vi "Main Loop.vi"(8 "error in (no error)":errorcluster, 10 "Chart Notifier":refnum<notifier>, 11 "Message Queues":T1) -> (0 "error out":errorcluster)   [LabVIEW 2018, in "4-20mA Module.lvlib" / "4-20mA Module Engine.lvlib"]
uses:
  4-20mA Module Engine.lvlib
  Pressure Regulator/Controls/4-20mA Message Queues.ctl
  support/Message Queue/Message Cluster.ctl
  State Cluster.ctl
  State Enum.ctl
  Pressure Transmitter/Pressure Transmitter Device Settings.ctl
  Pressure Reg Module/Pressure Regulator Device Settings.ctl
  Measure Instrument/PID 1 Parameters Cluster.ctl
  Pressure Regulator/Controls/4-20mA Display Cluster.ctl
  <vilib>/Platform/TimedLoop/XDataNode/timing_clust.ctl
  <vilib>/Platform/TimedLoop/XDataNode/nitl_modes.ctl
  <vilib>/Platform/TimedLoop/XDataNode/wakeup.ctl
  Tag VIs/Tag FGV Operation Enum.ctl
  Pressure Regulator/Controls/4-20mA Module Settings Cluster.ctl
  support/Message Queue/Enqueue Message (Single).vi
  <vilib>/Platform/TimedLoop/XDataNode/XDataNode.xnode
  support/Message Queue/Message Queue.lvlib
  <vilib>/Platform/TimedLoop/XDataNode/XDNodeRunTimeDep.lvlib
  Shared Variables/Dynamic Shared Variables.lvlib
  Pressure Transmitter/Pressure Transmitter Library.lvlib
  Pressure Reg Module/Pressure Regulator Library.lvlib
  Pressure Regulator/4-20mA Module.lvlib
  support/Support Library.lvlib
panel:
  out "Period (s)":dbl format="%_4g"
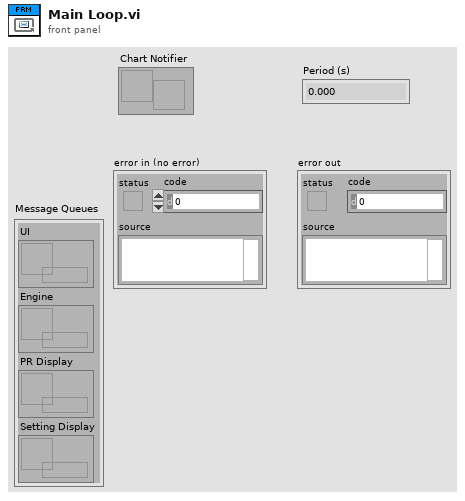
[diagram p1: front panel]
types:
  T1 = typedef "4-20mA Module.lvlib/4-20mA Message Queues.ctl" = cluster{"UI":refnum<queue>, "Engine":refnum<queue>, "PR Display":refnum<queue>, "Setting Display":refnum<queue>}
  T2 = typedef "4-20mA Module.lvlib/4-20mA Display Cluster.ctl" = cluster{"Input 4-20":dbl, "Output 4-20":dbl, "Cycle Period":dbl, "Status":enum16{"Off", "On", "Not Initialized"}}
  T3 = typedef "XDNodeRunTimeDep.lvlib/timing_clust.ctl" = cluster{"Expected End [f-1]":u64, "Actual End [f-1]":u64, "Finished Late? [f-1]":bool, "Expected End [i-1]":u64, "Actual End [i-1]":u64, "Finished Late? [i-1]":bool, "Expected Start [i]":u64, "Actual Start [i]":u64, "Expected Start [f]":u64, "Actual Start [f]":u64, "Source Name":string, "Structure Name":string, "Period":i64, "Deadline":i64, "Offset":i64, "Start":i64, "Priority":i32, "Timeout":i32, "Mode":T4, "Wakeup Reason":T5, "Error":errorcluster, "Source Type":string, "Secondary Source Type":string, "Global End Time":u64, "Global Start Time":u64, "Frame Duration":u64, "Iteration Duration":u64, "Assigned CPU":i32, "I/O Scan Engine Mode":u32}
  T4 = typedef "XDNodeRunTimeDep.lvlib/nitl_modes.ctl" = enum32{"No Change", "Process missed periods, maintain original phase", "Discard missed periods, maintain original phase", "Process missed periods, ignore original phase", "Discard missed periods, ignore original phase"}
  T5 = typedef "XDNodeRunTimeDep.lvlib/wakeup.ctl" = enum32{"Normal", "Aborted", "Asynchronous wakeup", "Timing source error", "Timed loop error", "Timeout"}
  T6 = cluster{"enable? (F)":bool, "name":string, "alarm on":bool, "priority":u32, "ack type":enum16{"Auto", "User", "None", "Each Occurrence"}, "area":string, "description":string, "log? (T)":bool}
  T7 = typedef "Tag FGV Operation Enum.ctl" = enum16{"Init", "Set Notification Queue", "Create Tag", "Commit", "Write Tag (Numeric)", "Write Tag (Boolean)", "Read All Tags", "Read One Tag", "Delete Tag Category", "Set Alarm Parameters (Numeric)", "Set Alarm Parameters (Boolean)", "Enable All Alarms", "Disable All Alarms", "Delete All Tags", "Read Alarms", "Ack Alarm", "Read Alarm Parameters (Numeric)", "Read Alarm Parameters (Boolean)"}
  T8 = enum32{"u32BitField", "bool", "double", "string", "int8", "uint8", "int16", "uint16", "int32", "uint32", "int64", "uint64", "single", "double waveform", "int16 waveform", "array of boolean", "array of int8", "array of uint8", "array of int16", "array of uint16", "array of int32", "array of uint32", "array of int64", "array of uint64", "array of single", "array of double", "array of double waveform", "array of int16 waveform", "array of string", "variant", "timestamp", "fixed point", "custom"}
  T9 = typedef "4-20mA Module.lvlib/4-20mA Module Engine.lvlib/State Enum.ctl" = enum16{"Measuring", "Idle", "Paused"}
  T10 = typedef "4-20mA Module.lvlib/4-20mA Module Settings Cluster.ctl" = cluster{"Cycle Period":dbl, "PID 2 Parameters":cluster{"Input Device":enum16{"Default", "4-20mA"}, "Output Device":enum16{"Default", "Equilibar Pressure Reg", "Flow Regulator"}, "Setpoint":dbl, "PID gains":cluster{"proportional gain (Kc)":dbl, "integral time (Ti, min)":dbl, "derivative time (Td, min)":dbl}, "output range":cluster{"output low":dbl, "output high":dbl}}, "Manual Entry":dbl, "Auto?":bool, "4-20mA Input Settings":T11, "4-20mA Out Settings":T12, "Input Channel Tag Name ":string}
  T11 = typedef "Pressure Transmitter Library.lvlib/Pressure Transmitter Device Settings.ctl" = cluster{"Input Channel ":u16}
  T12 = typedef "Pressure Regulator Library.lvlib/Pressure Regulator Device Settings.ctl" = cluster{"Output DAQ Task":refnum<k21>}
  T13 = typedef "4-20mA Module.lvlib/4-20mA Module Engine.lvlib/State Cluster.ctl" = cluster{"State":T9, "Start Time":timestamp, "Configuration":cluster{"Cycle Period":dbl, "PID 2 Parameters":cluster{"Input Device":enum16{"Default", "4-20mA"}, "Output Device":enum16{"Default", "Equilibar Pressure Reg", "Flow Regulator"}, "Setpoint":dbl, "PID gains":cluster{"proportional gain (Kc)":dbl, "integral time (Ti, min)":dbl, "derivative time (Td, min)":dbl}, "output range":cluster{"output low":dbl, "output high":dbl}}, "Manual Entry":dbl, "Auto?":bool, "4-20mA Input Settings":T11, "4-20mA Out Settings":T12, "Input Channel Tag Name ":string}, "Current Time":timestamp, "PID 1 Parameters":T14, "First Iteration":bool, "Data":cluster{"4-20mA Input":dbl, "PID 2 Process Variable":dbl, "PID 2 Output":dbl, "4-20mA Output":dbl}, "Process Name":string, "Pump On?":enum16{"Off", "On", "Not Initialized"}, "Input Error":bool, "Output Error":bool, "Log Started":bool, "Current Setpoint":dbl}
  T14 = typedef "PID 1 Parameters Cluster.ctl" = cluster{"Setpoint":dbl, "PID gains":cluster{"proportional gain (Kc)":dbl, "integral time (Ti, min)":dbl, "derivative time (Td, min)":dbl}}
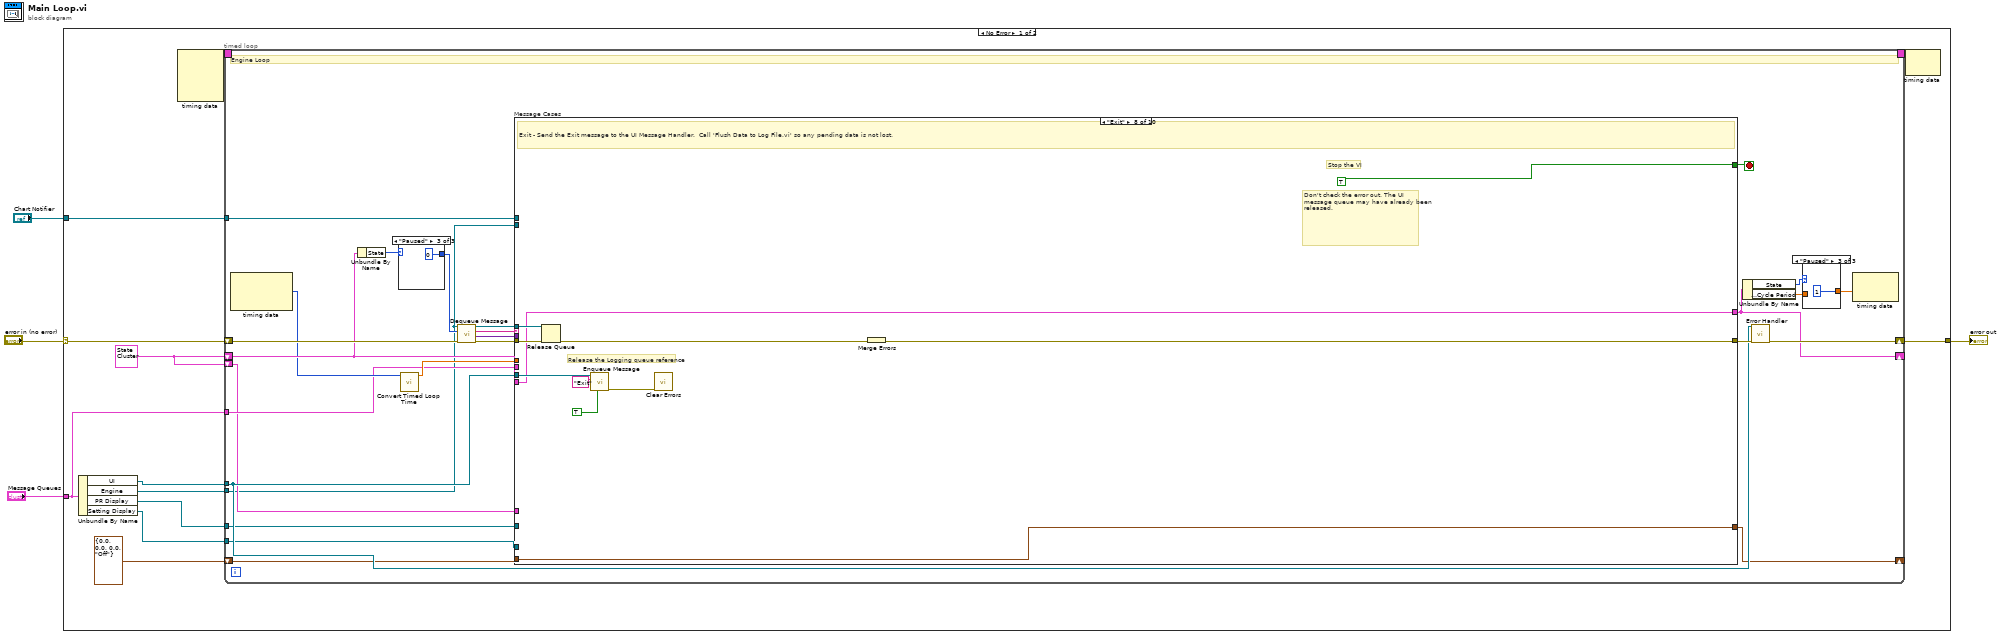
[diagram p0: block diagram]
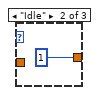
[diagram p3: hidden frame]
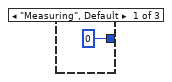
[diagram p4: hidden frame]
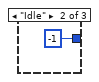
[diagram p5: hidden frame]
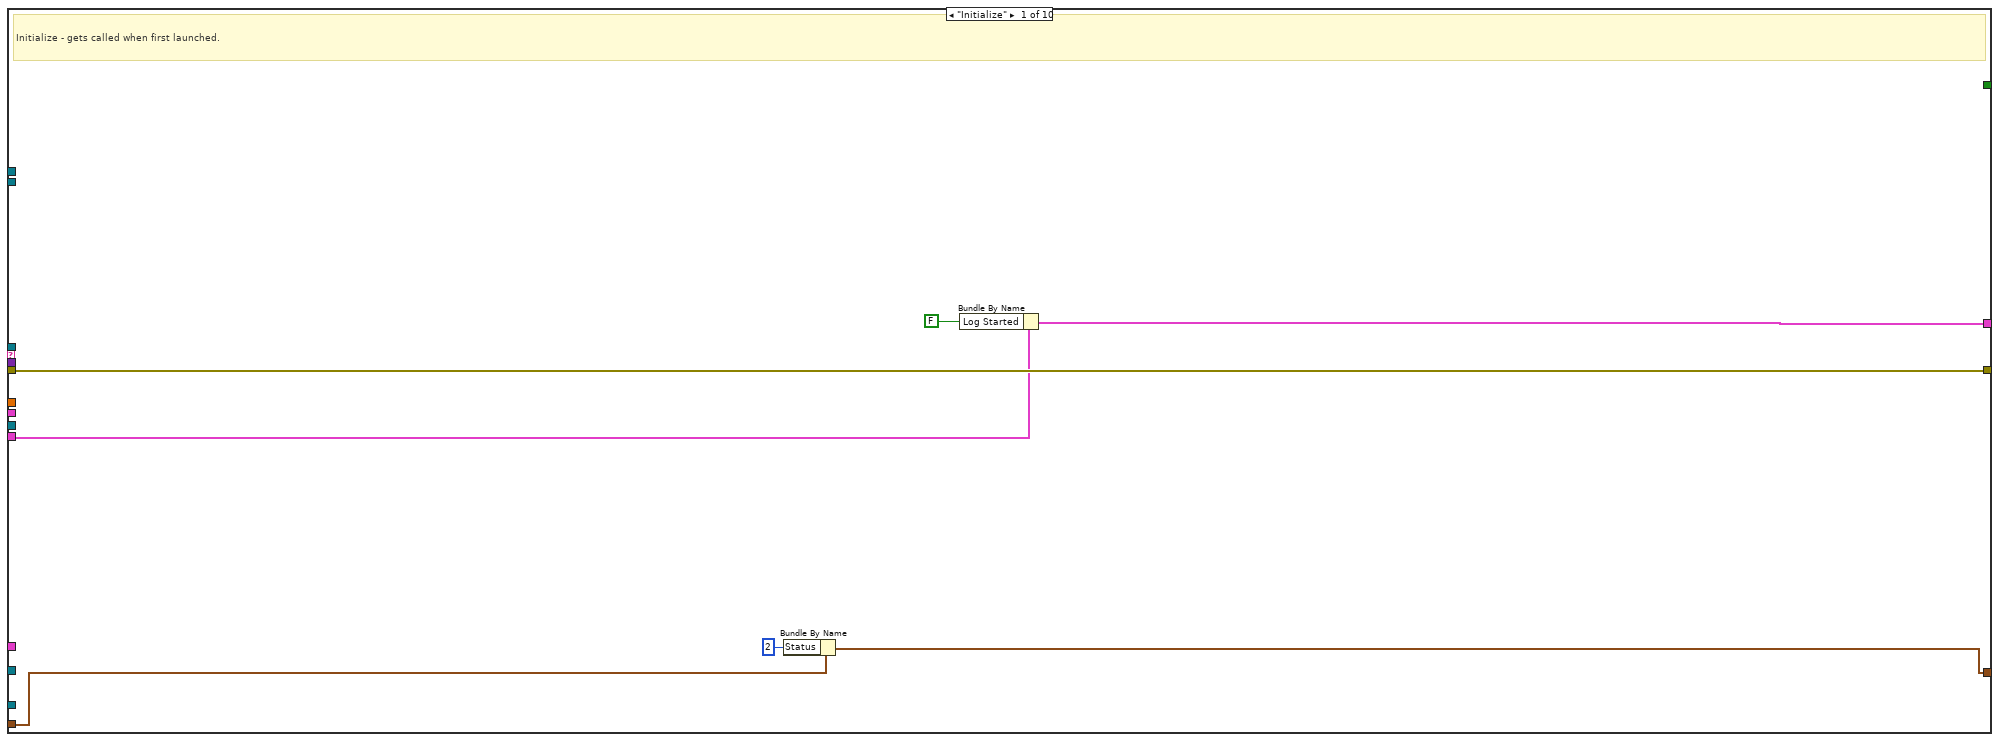
[diagram p6: hidden frame]
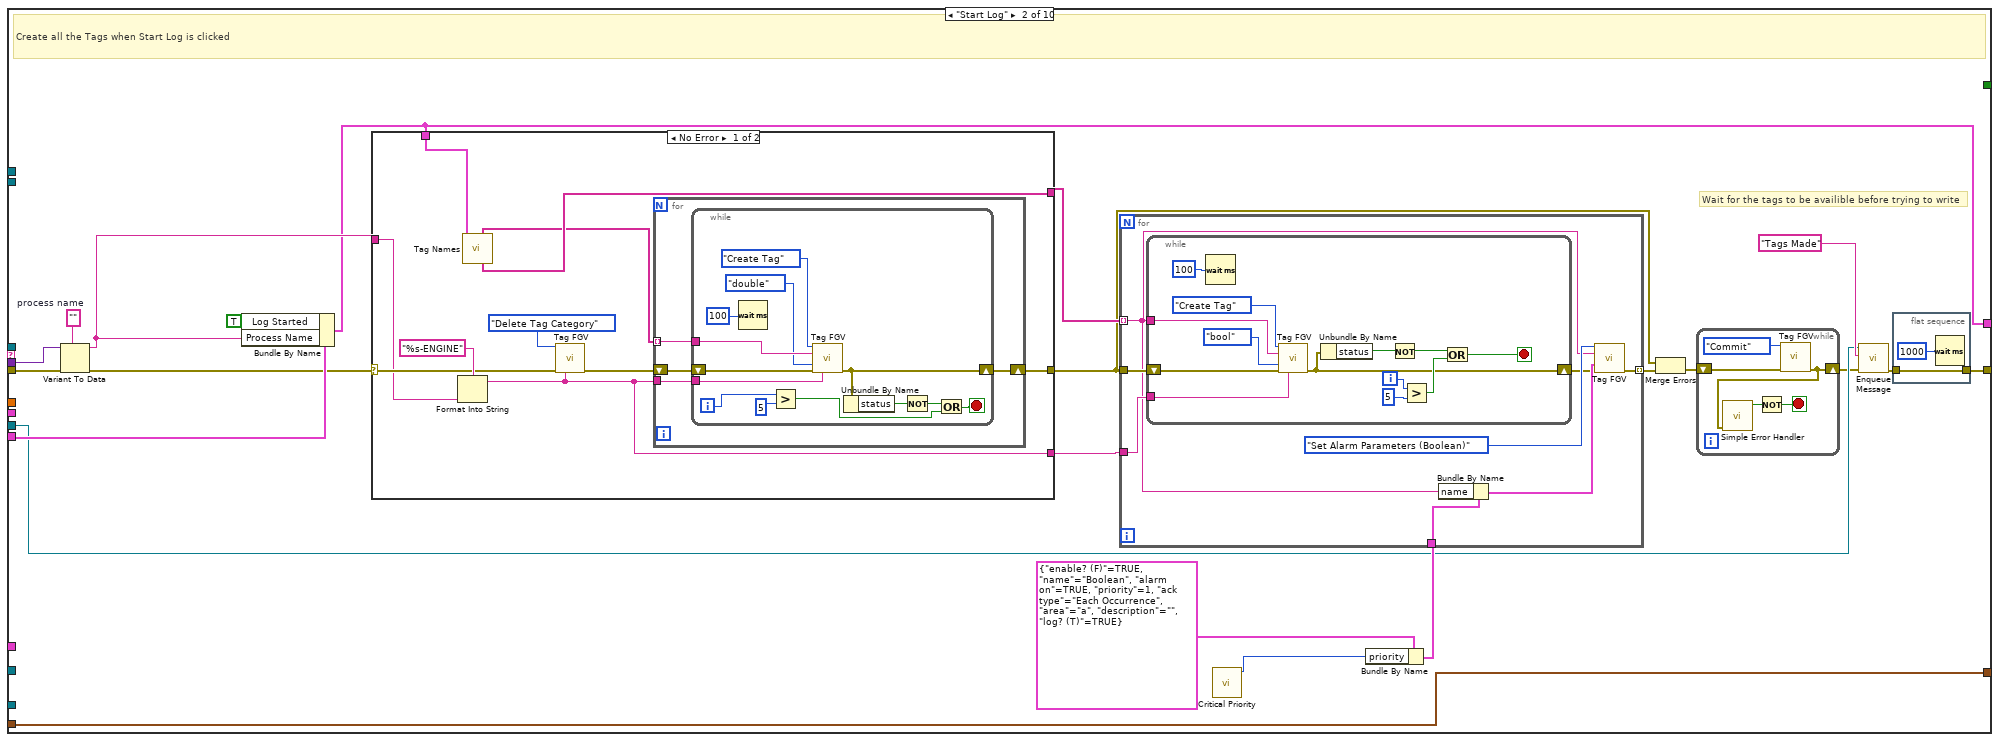
[diagram p7: hidden frame]
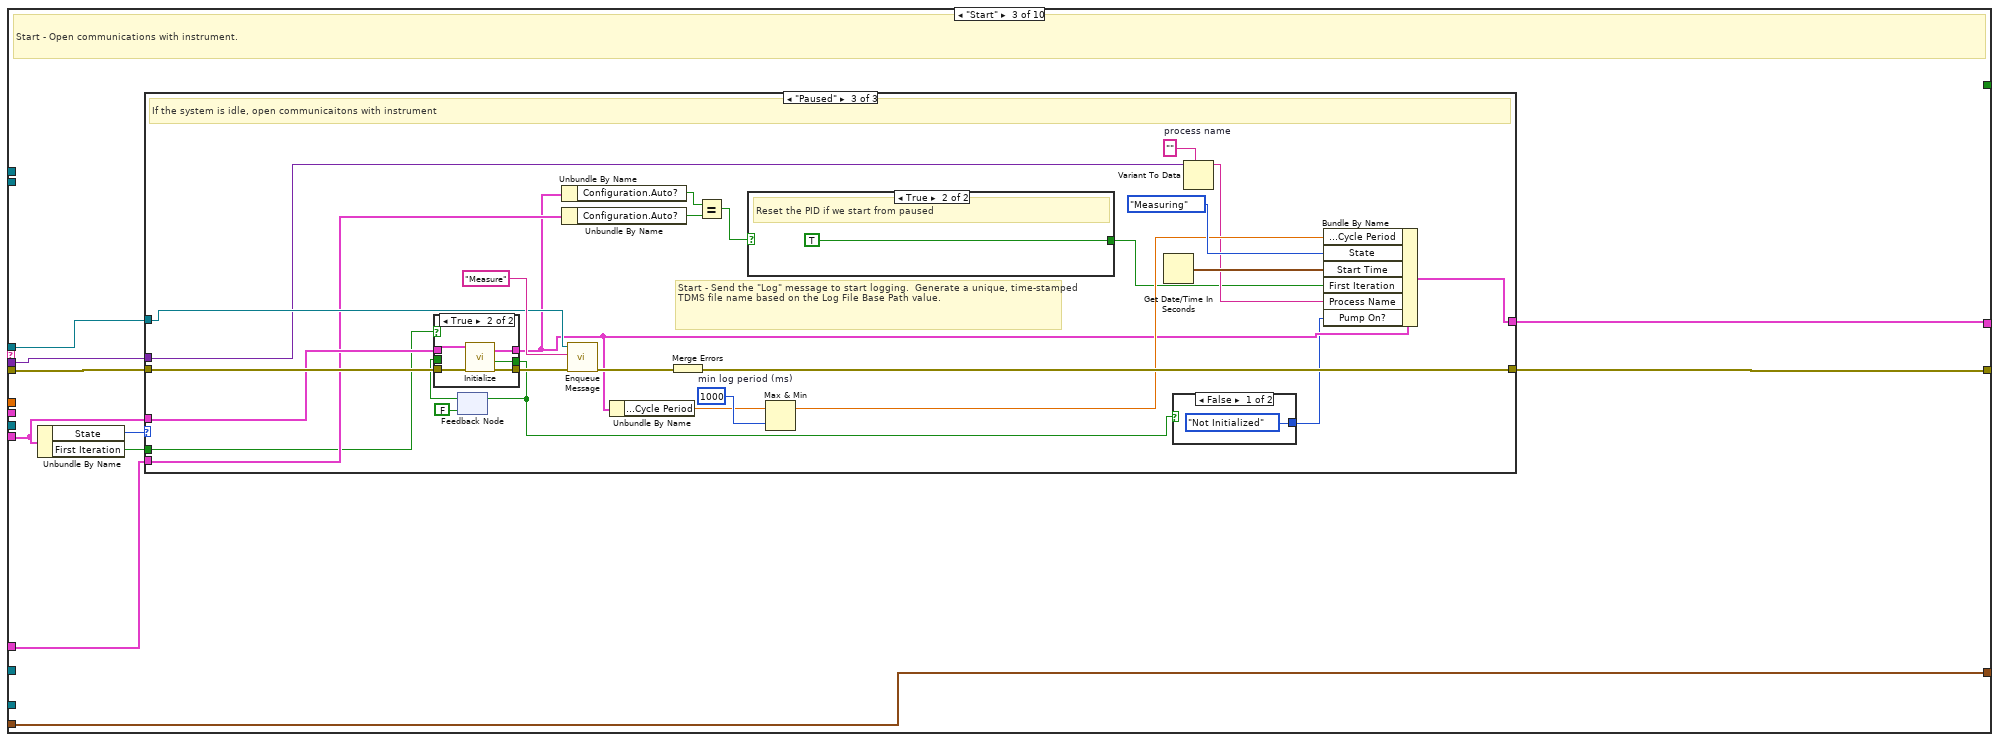
[diagram p9: hidden frame]
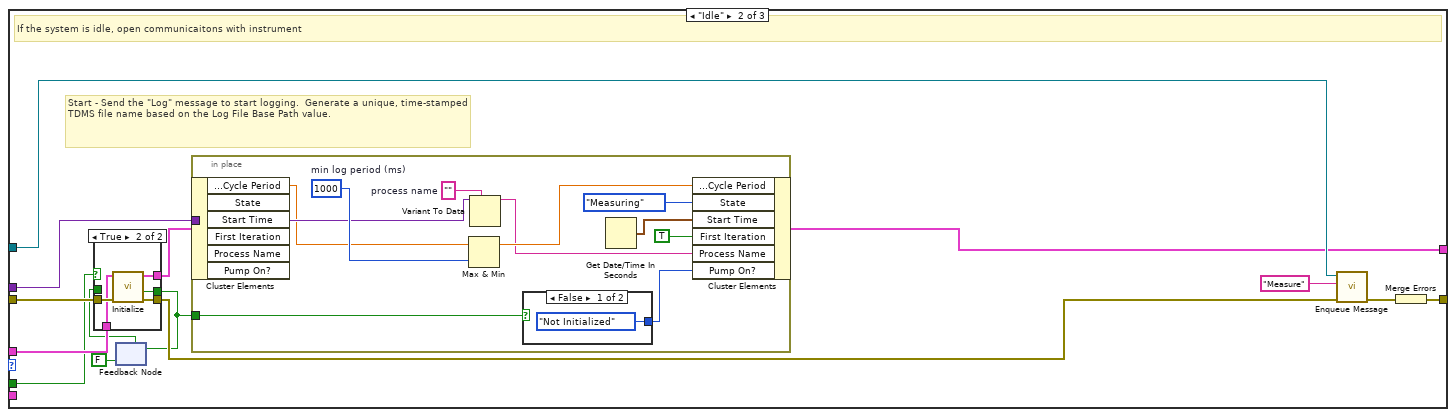
[diagram p11: hidden frame]
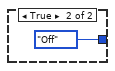
[diagram p12: hidden frame]
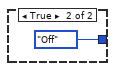
[diagram p15: hidden frame]
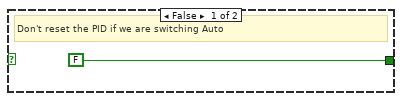
[diagram p16: hidden frame]
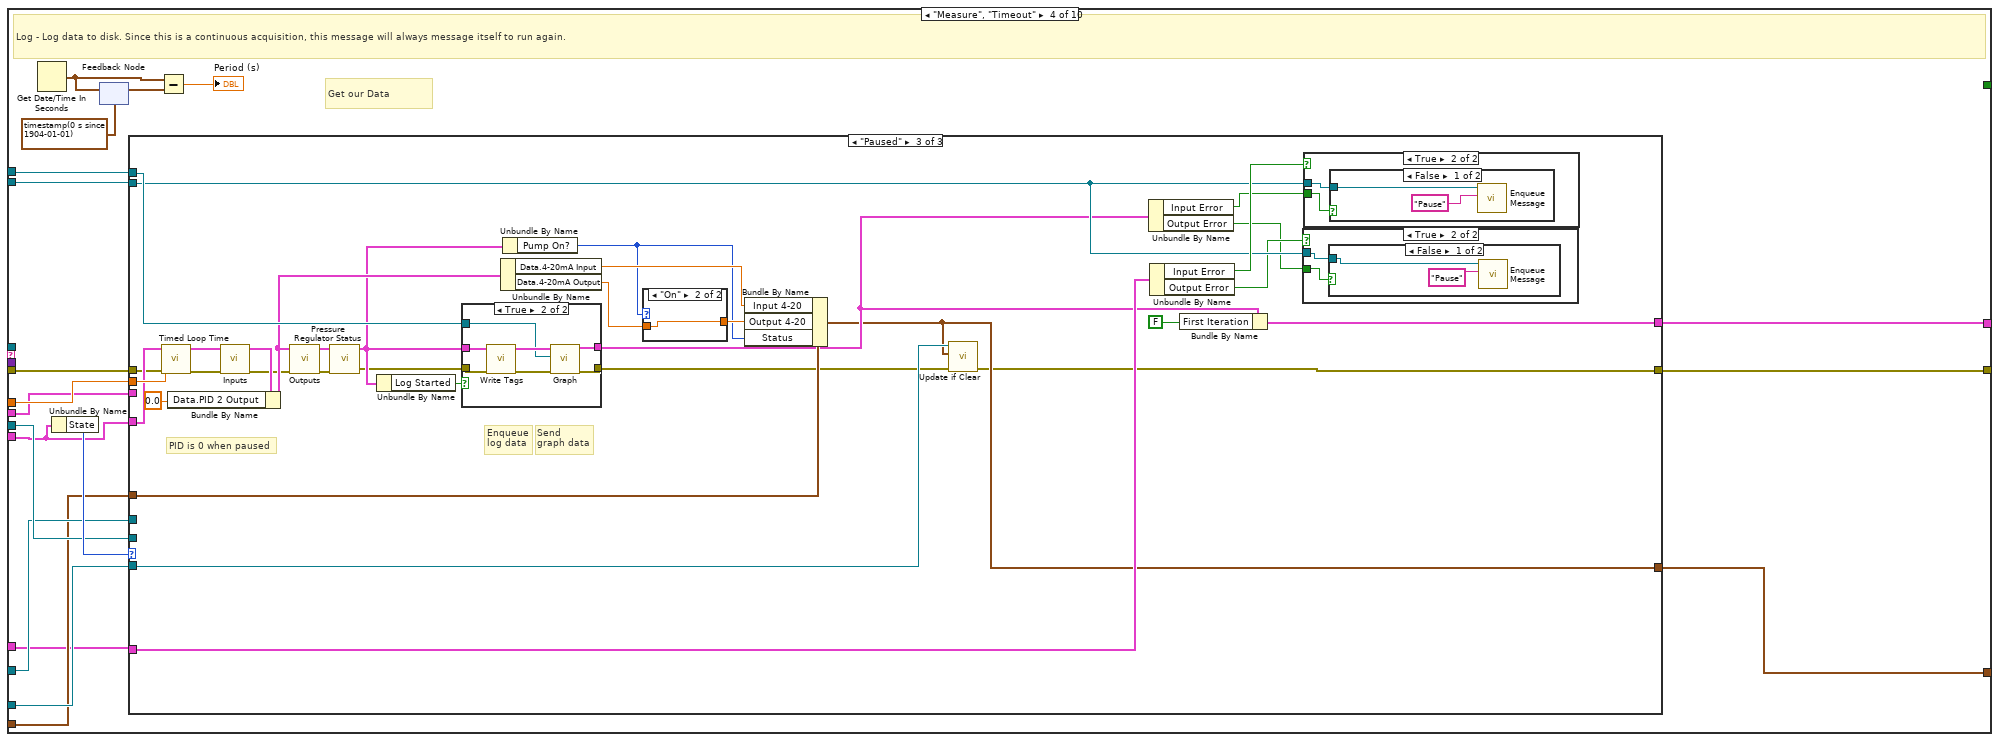
[diagram p17: hidden frame]
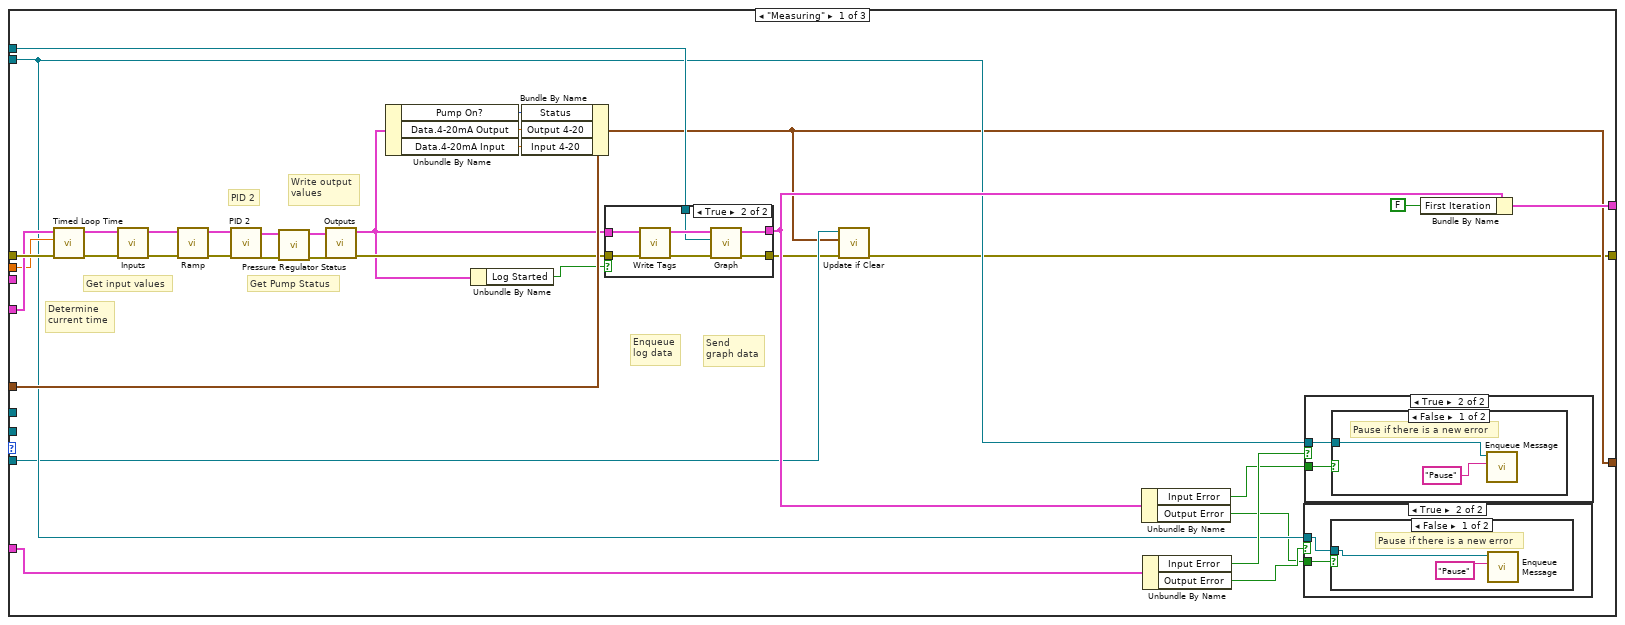
[diagram p18: hidden frame]
diagram:
  n1 = case shown="No Error" "error in (no error)" {
    selector: "error in (no error)" -> [w15 w453]
    tunnel: "Message Queues" -> [w11 _]
    tunnel: [w16 w453] -> w3
    tunnel: "Chart Notifier" -> [w9 _]
    frame No Error {
      w6 = T13 {"State"=enum."Idle", "Start Time"=timestamp(0 s since 1904-01-01), "Configuration"={"Cycle Period"=0.0, "PID 2 Parameters"={"Input Device"=enum."4-20mA", "Output Device"=enum."Equilibar Pressure Reg", "Setpoint"=0.0, "PID gains"={"proportional gain (Kc)"=1.0, "integral time (Ti, min)"=0.01, "derivative time (Td, min)"=0.0}, "output range"={"output low"=0.0, "output high"=100.0}}, "Manual Entry"=0.0, "Auto?"=TRUE, "4-20mA Input Settings"={"Input Channel "=0}, "4-20mA Out Settings"={"Output DAQ Task"=""}, "Input Channel Tag Name "=""}, "Current Time"=timestamp(0 s since 1904-01-01), "PID 1 Parameters"={"Setpoint"=0.0, "PID gains"={"proportional gain (Kc)"=1.0, "integral time (Ti, min)"=0.01, "derivative time (Td, min)"=0.0}}, "First Iteration"=FALSE, "Data"={"4-20mA Input"=0.0, "PID 2 Process Variable"=0.0, "PID 2 Output"=0.0, "4-20mA Output"=0.0}, "Process Name"="", "Pump On?"=enum."Off", "Input Error"=FALSE, "Output Error"=FALSE, "Log Started"=FALSE, "Current Setpoint"=0.0} ("State")
      n2 = Unbundle By Name(w11) -> ("UI"=w14:refnum<queue>, "Engine"=w10:refnum<queue>, "PR Display"=w8:refnum<queue>, "Setting Display"=w7:refnum<queue>)
      n3 = node-c288() -> (w13:T3)  [unwired: 4 in]
      n4 = timed-loop {
        tunnel: w10 -> [w19]
        shift-right: [w17] -> _
        shift-left: w6 -> [w34]
        shift-right: [w36] -> w16
        shift-left: w15 -> [w42]
        tunnel: w14 -> [w35]
        timing: w13 -> [_]
        timing-out: [_] -> w12
        tunnel: w11 -> [w26]
        tunnel: w9 -> [w25]
        tunnel: w8 -> [w24]
        tunnel: w7 -> [w23]
        shift-right: [w22] -> _
        shift-left: T2 {"Input 4-20"=0.0, "Output 4-20"=0.0, "Cycle Period"=0.0, "Status"=enum."Off"} ("PRM Display Cluster") -> [w18]
        shift-left: w6 -> [w21]
        stop <- w20 stop-if-true
        # "Engine Loop"
        n5 = node-c288() -> (w28:i64)  [unwired: 1 in, 2 out]
        n6 = Unbundle By Name(w34) -> ("State"=w33:T9)
        n7 = case shown="\"Idle\"" w33 {
          tunnel: [0 ("timeout in ms (-1)") -1 ("timeout in ms (-1)") 0 ("timeout in ms (-1)")] -> w32
          frame "Measuring", Default {
          }
          frame "Idle" {
          }
          frame "Paused" {
          }
        }
        n8 = call "Convert Timed Loop Time.vi"("Actual Start [i]"=w28) -> ("ET since start (s)"=w27:dbl)  [unwired: 10 in]
        n9 = call "Dequeue Message.vi"("error in (no error)"=w42, "timeout in ms (-1)"=w32, "Message Queue"=w19) -> ("error out"=w41:errorcluster, "Message Data"=w39:variant, "Message"=w40:string, "dup Message Queue"=w38:refnum<queue>)  [unwired: 5 in]
        n10 = case "Message Cases" shown="\"Exit\"" w40 {
          selector: w40 -> [_ _ _ _ _ _ _ _ _ w447]
          tunnel: w38 -> [_ _ w147 _ w365 _ _ w432 _ _]
          tunnel: w41 -> [w60 w79 w146 w240 w362 w384 w426 w435 w442 _]
          tunnel: [w60 w62 w148 w241 w355 w377 w424 w437 w441 w443] -> w37
          tunnel: w34 -> [w59 w78 w143 w239 w361 w386 w423 w428 w439 w449]
          tunnel: [_ _ _ _ _ _ _ TRUE _ _] -> w20
          tunnel: w39 -> [_ w80 w144 _ _ _ w427 _ _ _]
          tunnel: w35 -> [_ w67 _ w242 w364 w388 _ w436 _ _]
          tunnel: w27 -> [_ _ _ w238 _ _ _ _ _ _]
          tunnel: w26 -> [_ _ _ w237 _ _ _ _ _ _]
          tunnel: w25 -> [_ _ _ w233 _ _ _ _ _ _]
          tunnel: w24 -> [_ _ _ w232 w360 _ _ _ _ _]
          tunnel: w23 -> [_ _ _ w231 w358 w380 _ _ _ _]
          tunnel: w18 -> [w56 w82 w142 w230 w357 w379 w425 w429 w440 w450]
          tunnel: [w54 w82 w142 w229 w357 w379 w425 w429 w440 w450] -> w22
          tunnel: w21 -> [_ _ w141 w228 _ _ _ _ _ _]
          tunnel: w19 -> [_ _ _ w227 _ _ _ _ _ _]
          tunnel: [w57 w66 w139 w226 w359 w381 w420 w428 w439 w449] -> w17
          frame "Initialize" {
            # "Initialize - gets called when first launched."
            n11 = Bundle By Name(cluster=w56, "Status"=u16 2) -> (w54:T2)
            n12 = Bundle By Name(cluster=w59, "Log Started"=FALSE) -> (w57:T13)
          }
          frame "Start Log" {
            w81 = ""  # process name
            # "Wait for the tags to be availible before trying to write"
            # "Create all the Tags when Start Log is clicked"
            n13 = Variant To Data(error in=w79, type=w81, Variant=w80) -> (data=w76:string, error out=w77:errorcluster)
            n14 = Bundle By Name(cluster=w78, "Log Started"=TRUE, "Process Name"=w76) -> (w66:T13)
            n15 = case shown="No Error" w77 {
              selector: w77 -> [w117 w138]
              tunnel: [w120 w138] -> w61
              tunnel: w76 -> [w115 _]
              tunnel: [w114 _] -> w72
              tunnel: [w113 _] -> w70
              tunnel: w66 -> [w112 _]
              frame No Error {
                n16 = Format Into String(format string="%s-ENGINE", w115) -> (resulting string=w113:string)  [unwired: 2 in, 1 out]
                n17 = call "Tag Names.vi"("State in"=w112) -> ("All Boolean Tags"=w114:string[], "All  Numeric Tags"=w111:string[])  [unwired: 8 in, 1 out]
                n18 = call "Tag FGV.vi"("Operation"=Tag_FGV_Operation_Enum."Delete Tag Category", "error in (no error)"=w117, "Tag Category"=w113) -> ("error out"=w116:errorcluster)  [unwired: 5 in, 7 out]
                n19 = for {
                  tunnel: w111 -> [w124] mode=indexing
                  shift-right: [w122] -> w120
                  shift-left: w116 -> [w123]
                  tunnel: w113 -> [w121]
                  n20 = while {
                    tunnel: w124 -> [w136]
                    tunnel: w121 -> [w133]
                    shift-right: [w132] -> w122
                    shift-left: w123 -> [w134]
                    i -> [w127]
                    stop <- w125 stop-if-true
                    n21 = Wait (ms)(milliseconds to wait=u32 100) -> ()  [unwired: 1 out]
                    n22 = Greater?(x=w127, y=5 ("x")) -> (0:w126:bool)
                    n23 = call "Tag FGV.vi"("Operation"=Tag_FGV_Operation_Enum."Create Tag", "Tag Name"=w136, "Data"=T8."double" ("data type"), "error in (no error)"=w134, "Tag Category"=w133) -> ("error out"=w132:errorcluster)  [unwired: 3 in, 7 out]
                    n24 = Unbundle By Name(w132) -> ("status"=w131:bool)
                    n25 = Not(x=w131) -> (.not. x?=w129:bool)
                    n26 = Or(x=w129, y=w126) -> (x .or. y?=w125:bool)
                  }
                }
              }
              frame Error {
              }
            }
            n27 = call "Critical Priority.vi"() -> ("critical priority"=w74:i32)  [unwired: 11 in]
            n28 = Bundle By Name(cluster=T6 {"enable? (F)"=TRUE, "name"="Boolean", "alarm on"=TRUE, "priority"=1, "ack type"=enum."Each Occurrence", "area"="a", "description"="", "log? (T)"=TRUE} ("Boolean alarm settings"), "priority"=w74) -> (w73:T6)
            n29 = for {
              tunnel: w73 -> [w97]
              tunnel: [w96] -> w71 mode=indexing
              tunnel: w72 -> [w90] mode=indexing
              tunnel: w61 -> [w92]
              tunnel: w70 -> [w93]
              n30 = while {
                tunnel: w90 -> [w109]
                tunnel: w93 -> [w106]
                shift-right: [w98] -> w91
                shift-left: w92 -> [w107]
                i -> [w101]
                stop <- w99 stop-if-true
                n31 = Wait (ms)(milliseconds to wait=u32 100) -> ()  [unwired: 1 out]
                n32 = call "Tag FGV.vi"("Operation"=Tag_FGV_Operation_Enum."Create Tag", "Tag Name"=w109, "Data"=T8."bool" ("data type"), "error in (no error)"=w107, "Tag Category"=w106) -> ("error out"=w98:errorcluster)  [unwired: 3 in, 7 out]
                n33 = Unbundle By Name(w98) -> ("status"=w105:bool)
                n34 = Not(x=w105) -> (.not. x?=w103:bool)
                n35 = Greater?(x=w101, y=5 ("x")) -> (0:w100:bool)
                n36 = Or(x=w103, y=w100) -> (x .or. y?=w99:bool)
              }
              n37 = Bundle By Name(cluster=w97, "name"=w90) -> (w95:T6)
              n38 = call "Tag FGV.vi"("Operation"=Tag_FGV_Operation_Enum."Set Alarm Parameters (Boolean)", "Tag Name"=w90, "Data"=w95, "error in (no error)"=w91) -> ("error out"=w96:errorcluster)  [unwired: 4 in, 7 out]
            }
            n39 = Merge Errors(w61, w71) -> (w65:errorcluster)
            n40 = while {
              shift-right: [w87] -> w64
              shift-left: w65 -> [w88]
              stop <- w85 stop-if-true
              n41 = call "Tag FGV.vi"("Operation"=Tag_FGV_Operation_Enum."Commit", "error in (no error)"=w88) -> ("error out"=w87:errorcluster)  [unwired: 6 in, 7 out]
              n42 = call <vilib>:"Simple Error Handler.vi"("error in (no error)"=w87) -> ("error?"=w86:bool)  [unwired: 4 in, 4 out]
              n43 = Not(x=w86) -> (.not. x?=w85:bool)
            }
            n44 = call-poly "Enqueue Message.vi"("error in (no error)"=w64, "Message"="Tags Made", "Message Queue"=w67) -> ("error out"=w63:errorcluster)  [unwired: 7 in, 1 out]
            n45 = flat-sequence {
              tunnel: [w83] -> w62
              tunnel: w63 -> [w83]
              frame #0 {
                n46 = Wait (ms)(milliseconds to wait=u32 1000) -> ()  [unwired: 1 out]
              }
            }
          }
          frame "Start" {
            # "Start - Open communications with instrument."
            n47 = Unbundle By Name(w143) -> ("State"=w145:T9, "First Iteration"=w140:bool)
            n48 = case shown="\"Paused\"" w145 {
              tunnel: [w149 w164 w212] -> w148
              tunnel: w147 -> [_ w161 w203]
              tunnel: w146 -> [w149 w160 w201]
              tunnel: w143 -> [w150 w159 w200]
              tunnel: [w150 w152 w210] -> w139
              tunnel: w144 -> [_ w158 w198]
              tunnel: w141 -> [_ _ w194]
              tunnel: w140 -> [_ w154 w189]
              frame "Measuring", Default {
                # "The system is already running. Ignore the \"Start\" message."
              }
              frame "Idle" {
                # "Start - Send the \"Log\" message to start logging.  Generate a unique, time-stamped TDMS file name based on the Log File Base Path value."
                # "If the system is idle, open communicaitons with instrument"
                n49 = feedback #1(FALSE ("Pump Initialized")) -> (w156:bool)
                n50 = case shown="True" w154 {
                  tunnel: w160 -> [w179 w185]
                  tunnel: w159 -> [w180 w184]
                  tunnel: [w180 w183] -> w153
                  tunnel: [w179 w182] -> w157
                  tunnel: [w178 w181] -> w155
                  tunnel: w156 -> [w178 _]
                  frame False {
                  }
                  frame True {
                    n51 = call "Initialize.vi"("error in (no error)"=w185, "State in"=w184) -> ("error out"=w182:errorcluster, "Pump Initialized"=w181:bool, "State out"=w183:T13)  [unwired: 7 in]
                  }
                }
                n52 = feedback-in #1(w155) -> ()
                n53 = in-place {
                  in-place-border: w158 -> [w173]
                  in-place-border: w155 -> [w172]
                  w174 = ""  # process name
                  w175 = 1000  # min log period (ms)
                  n54 = in-place-cluster #2(w153) -> ("Configuration.Cycle Period"=w171:dbl)  [unwired: 5 out]
                  n55 = Max & Min(x=w171, y=w175) -> (max(x,y)=w170:dbl)  [unwired: 1 out]
                  n56 = Variant To Data(type=w174, Variant=w173) -> (data=w166:string)  [unwired: 1 in, 1 out]
                  n57 = case shown="False" w172 {
                    tunnel: [enum16{"Off", "On", "Not Initialized"}."Not Initialized" ("Pump On?") enum16{"Off", "On", "Not Initialized"}."Off" ("Pump On?")] -> w165
                    frame False {
                    }
                    frame True {
                    }
                  }
                  n58 = Get Date/Time In Seconds() -> (seconds since 1Jan1904=w168:timestamp)
                  n59 = in-place-cluster #2("Configuration.Cycle Period"=w170, "State"=State_Enum."Measuring", "Start Time"=w168, "First Iteration"=TRUE, "Process Name"=w166, "Pump On?"=w165) -> (w152:T13)
                }
                n60 = call-poly "Enqueue Message.vi"("error in (no error)"=w157, "Message"="Measure", "Message Queue"=w161) -> ("error out"=w162:errorcluster)  [unwired: 7 in, 1 out]
                n61 = Merge Errors(w162) -> (w164:errorcluster)
              }
              frame "Paused" {
                w199 = ""  # process name
                w207 = 1000  # min log period (ms)
                # "Start - Send the \"Log\" message to start logging.  Generate a unique, time-stamped TDMS file name based on the Log File Base Path value."
                # "If the system is idle, open communicaitons with instrument"
                n62 = feedback #3(FALSE ("Pump Initialized")) -> (w188:bool)
                n63 = case shown="True" w189 {
                  tunnel: [w215 w220] -> w202
                  tunnel: w201 -> [w215 w219]
                  tunnel: w200 -> [w214 w218]
                  tunnel: [w214 w217] -> w191
                  tunnel: [w213 w216] -> w187
                  tunnel: w188 -> [w213 _]
                  frame False {
                  }
                  frame True {
                    n64 = call "Initialize.vi"("error in (no error)"=w219, "State in"=w218) -> ("error out"=w220:errorcluster, "Pump Initialized"=w216:bool, "State out"=w217:T13)  [unwired: 7 in]
                  }
                }
                n65 = feedback-in #3(w187) -> ()
                n66 = Unbundle By Name(w191) -> ("Configuration.Auto?"=w195:bool)
                n67 = Unbundle By Name(w194) -> ("Configuration.Auto?"=w193:bool)
                n68 = call-poly "Enqueue Message.vi"("error in (no error)"=w202, "Message"="Measure", "Message Queue"=w203) -> ("error out"=w208:errorcluster)  [unwired: 7 in, 1 out]
                n69 = Unbundle By Name(w191) -> ("Configuration.Cycle Period"=w206:dbl)
                n70 = Merge Errors(w208) -> (w212:errorcluster)
                n71 = Equal?(x=w195, y=w193) -> (x = y?=w196:bool)
                n72 = case shown="True" w196 {
                  tunnel: [FALSE ("First Iteration") TRUE ("First Iteration")] -> w192
                  frame False {
                    # "Don't reset the PID if we are switching Auto"
                  }
                  frame True {
                    # "Reset the PID if we start from paused"
                  }
                }
                n73 = Max & Min(x=w206, y=w207) -> (max(x,y)=w205:dbl)  [unwired: 1 out]
                n74 = Get Date/Time In Seconds() -> (seconds since 1Jan1904=w204:timestamp)
                n75 = case shown="False" w187 {
                  tunnel: [enum16{"Off", "On", "Not Initialized"}."Not Initialized" ("Pump On?") enum16{"Off", "On", "Not Initialized"}."Off" ("Pump On?")] -> w190
                  frame False {
                  }
                  frame True {
                  }
                }
                n76 = Variant To Data(type=w199, Variant=w198) -> (data=w197:string)  [unwired: 1 in, 1 out]
                n77 = Bundle By Name(cluster=w191, "Configuration.Cycle Period"=w205, "State"=State_Enum."Measuring", "Start Time"=w204, "First Iteration"=w192, "Process Name"=w197, "Pump On?"=w190) -> (w210:T13)
              }
            }
          }
          frame "Measure", "Timeout" {
            # "Get our Data"
            # "Log - Log data to disk. Since this is a continuous acquisition, this message will always message itself to run again."
            n78 = Get Date/Time In Seconds() -> (seconds since 1Jan1904=w235:timestamp)
            n79 = Unbundle By Name(w239) -> ("State"=w243:T9)
            n80 = feedback-in #4(w235) -> ()
            n81 = feedback #4(timestamp(0 s since 1904-01-01) ("seconds since 1Jan1904")) -> (w236:timestamp)
            n82 = case shown="\"Idle\", Default" w243 {
              tunnel: w240 -> [w277 w299 w321]
              tunnel: w239 -> [w276 w301 w322]
              tunnel: w242 -> [_ _ _]
              tunnel: [w244 w296 w302] -> w241
              tunnel: [w274 w301 w320] -> w226
              tunnel: w238 -> [w275 _ w333]
              tunnel: w237 -> [_ _ _]
              tunnel: w233 -> [w272 _ w334]
              tunnel: w232 -> [_ w300 _]
              tunnel: w231 -> [w247 w298 w305]
              tunnel: w230 -> [w271 w295 w332]
              tunnel: [w246 w295 w304] -> w229
              tunnel: w228 -> [w254 _ w329]
              tunnel: w227 -> [w267 _ w326]
              frame "Measuring" {
                # "Get Pump Status"
                # "Send\ngraph data"
                # "Enqueue\nlog data"
                # "PID 2"
                # "Determine\ncurrent time"
                # "Write output\nvalues"
                # "Get input values"
                n83 = call "Timed Loop Time.vi"("error in (no error)"=w277, "ET since start (s)"=w275, "State in"=w276) -> ("error out"=w255:errorcluster, "State out"=w256:T13)  [unwired: 7 in]
                n84 = call "Inputs.vi"("error in (no error)"=w255, "State in"=w256) -> ("error out"=w251:errorcluster, "State out"=w253:T13)  [unwired: 8 in]
                n85 = call "Ramp.vi"("error in (no error)"=w251, "New State"=w253) -> ("error out"=w250:errorcluster, "State"=w252:T13)  [unwired: 8 in]
                n86 = call "PID 2.vi"("error in (no error)"=w250, "State in"=w252) -> ("error out"=w260:errorcluster, "State out"=w261:T13)  [unwired: 8 in]
                n87 = call "Pressure Regulator Status.vi"("error in (no error)"=w260, "State In"=w261) -> ("error out"=w259:errorcluster, "State Out"=w258:T13)  [unwired: 8 in]
                n88 = call "Outputs.vi"("error in (no error)"=w259, "State in"=w258) -> ("error out"=w262:errorcluster, "State out"=w257:T13)  [unwired: 8 in]
                n89 = Unbundle By Name(w257) -> ("Pump On?"=w249:enum16{"Off", "On", "Not Initialized"}, "Data.4-20mA Output"=w263:dbl, "Data.4-20mA Input"=w248:dbl)
                n90 = Unbundle By Name(w257) -> ("Log Started"=w264:bool)
                n91 = Bundle By Name(cluster=w271, "Status"=w249, "Output 4-20"=w263, "Input 4-20"=w248) -> (w246:T2)
                n92 = case shown="True" w264 {
                  tunnel: [w279 w284] -> w245
                  tunnel: w272 -> [_ w283]
                  tunnel: w257 -> [w278 w282]
                  tunnel: w262 -> [w279 w281]
                  tunnel: [w278 w280] -> w268
                  frame False {
                  }
                  frame True {
                    n93 = call "Write Tags.vi"("error in (no error)"=w281, "State in"=w282) -> ("error out"=w285:errorcluster, "State out"=w286:T13)  [unwired: 8 in]
                    n94 = call "Graph.vi"("error in (no error)"=w285, "notifier out"=w283, "State in"=w286) -> ("error out"=w284:errorcluster, "State out"=w280:T13)  [unwired: 7 in]
                  }
                }
                n95 = call "Update if Clear.vi"("error in (no error)"=w245, "Message Data"=w246, "Queue in"=w247) -> ("error out"=w244:errorcluster)  [unwired: 8 in]
                n96 = Unbundle By Name(w268) -> ("Input Error"=w269:bool, "Output Error"=w265:bool)
                n97 = Unbundle By Name(w254) -> ("Input Error"=w270:bool, "Output Error"=w266:bool)
                n98 = case shown="True" w266 {
                  tunnel: w265 -> [_ w288]
                  tunnel: w267 -> [_ w287]
                  frame False {
                  }
                  frame True {
                    n99 = case shown="False" w288 {
                      tunnel: w287 -> [w290 _]
                      frame False {
                        # "Pause if there is a new error"
                        n100 = call-poly "Enqueue Message.vi"("Message"="Pause", "Message Queue"=w290) -> ()  [unwired: 8 in, 2 out]
                      }
                      frame True {
                      }
                    }
                  }
                }
                n101 = case shown="True" w270 {
                  tunnel: w269 -> [_ w292]
                  tunnel: w267 -> [_ w291]
                  frame False {
                  }
                  frame True {
                    n102 = case shown="False" w292 {
                      tunnel: w291 -> [w294 _]
                      frame False {
                        # "Pause if there is a new error"
                        n103 = call-poly "Enqueue Message.vi"("Message"="Pause", "Message Queue"=w294) -> ()  [unwired: 8 in, 2 out]
                      }
                      frame True {
                      }
                    }
                  }
                }
                n104 = Bundle By Name(cluster=w268, "First Iteration"=FALSE) -> (w274:T13)
              }
              frame "Idle", Default {
                n105 = call "Update if Clear.vi"("error in (no error)"=w299, "Message Data"=w295, "Queue in"=w300) -> ("error out"=w297:errorcluster)  [unwired: 8 in]
                n106 = call "Update if Clear.vi"("error in (no error)"=w297, "Message Data"=w295, "Queue in"=w298) -> ("error out"=w296:errorcluster)  [unwired: 8 in]
              }
              frame "Paused" {
                # "PID is 0 when paused"
                # "Send\ngraph data"
                # "Enqueue\nlog data"
                n107 = call "Timed Loop Time.vi"("error in (no error)"=w321, "ET since start (s)"=w333, "State in"=w322) -> ("error out"=w309:errorcluster, "State out"=w311:T13)  [unwired: 7 in]
                n108 = call "Inputs.vi"("error in (no error)"=w309, "State in"=w311) -> ("error out"=w308:errorcluster, "State out"=w310:T13)  [unwired: 8 in]
                n109 = Bundle By Name(cluster=w310, "Data.PID 2 Output"=0.0 ("Data.PID 2 output")) -> (w318:T13)
                n110 = call "Outputs.vi"("error in (no error)"=w308, "State in"=w318) -> ("error out"=w314:errorcluster, "State out"=w307:T13)  [unwired: 8 in]
                n111 = call "Pressure Regulator Status.vi"("error in (no error)"=w314, "State In"=w307) -> ("error out"=w312:errorcluster, "State Out"=w313:T13)  [unwired: 8 in]
                n112 = Unbundle By Name(w313) -> ("Log Started"=w317:bool)
                n113 = case shown="True" w317 {
                  tunnel: w334 -> [_ w341]
                  tunnel: [w335 w340] -> w303
                  tunnel: w313 -> [w336 w339]
                  tunnel: w312 -> [w335 w338]
                  tunnel: [w336 w337] -> w315
                  frame False {
                  }
                  frame True {
                    n114 = call "Write Tags.vi"("error in (no error)"=w338, "State in"=w339) -> ("error out"=w343:errorcluster, "State out"=w342:T13)  [unwired: 8 in]
                    n115 = call "Graph.vi"("error in (no error)"=w343, "notifier out"=w341, "State in"=w342) -> ("error out"=w340:errorcluster, "State out"=w337:T13)  [unwired: 7 in]
                  }
                }
                n116 = Unbundle By Name(w318) -> ("Data.4-20mA Input"=w316:dbl, "Data.4-20mA Output"=w331:dbl)
                n117 = Unbundle By Name(w313) -> ("Pump On?"=w306:enum16{"Off", "On", "Not Initialized"})
                n118 = case shown="\"On\"" w306 {
                  tunnel: w331 -> [_ w353]
                  tunnel: [0.0 w353] -> w330
                  frame "Off", Default {
                  }
                  frame "On" {
                  }
                }
                n119 = Bundle By Name(cluster=w332, "Input 4-20"=w316, "Output 4-20"=w330, "Status"=w306) -> (w304:T2)
                n120 = call "Update if Clear.vi"("error in (no error)"=w303, "Message Data"=w304, "Queue in"=w305) -> ("error out"=w302:errorcluster)  [unwired: 8 in]
                n121 = Unbundle By Name(w315) -> ("Input Error"=w327:bool, "Output Error"=w324:bool)
                n122 = Unbundle By Name(w329) -> ("Input Error"=w328:bool, "Output Error"=w325:bool)
                n123 = Bundle By Name(cluster=w315, "First Iteration"=FALSE) -> (w320:T13)
                n124 = case shown="True" w325 {
                  tunnel: w324 -> [_ w345]
                  tunnel: w326 -> [_ w344]
                  frame False {
                  }
                  frame True {
                    n125 = case shown="False" w345 {
                      tunnel: w344 -> [w347 _]
                      frame False {
                        n126 = call-poly "Enqueue Message.vi"("Message"="Pause", "Message Queue"=w347) -> ()  [unwired: 8 in, 2 out]
                      }
                      frame True {
                      }
                    }
                  }
                }
                n127 = case shown="True" w328 {
                  tunnel: w327 -> [_ w349]
                  tunnel: w326 -> [_ w348]
                  frame False {
                  }
                  frame True {
                    n128 = case shown="False" w349 {
                      tunnel: w348 -> [w351 _]
                      frame False {
                        n129 = call-poly "Enqueue Message.vi"("Message"="Pause", "Message Queue"=w351) -> ()  [unwired: 8 in, 2 out]
                      }
                      frame True {
                      }
                    }
                  }
                }
              }
            }
            n130 = Subtract(x=w235, y=w236) -> (x-y=→"Period (s)":dbl)
          }
          frame "Stop" {
            # "Stop - Flush the message queue of any pending \"Log\" messages. Call 'Flush Data to Log File.vi' so any pending data is not lost."
            n131 = Unbundle By Name(w361) -> ("State"=w363:T9)
            n132 = case shown="\"Measuring\", Default" w363 {
              tunnel: [w370 w376] -> w354
              tunnel: w362 -> [w366 w376]
              tunnel: w365 -> [_ _]
              tunnel: w364 -> [w374 _]
              tunnel: w361 -> [w368 w375]
              tunnel: [w372 w375] -> w359
              frame "Measuring", Default {
                # "If the system is logging, stop logging."
                n133 = call "Close.vi"("error in (no error)"=w366, "State in"=w368) -> ("error out"=w367:errorcluster, "State out"=w369:T13)  [unwired: 8 in]
                n134 = Bundle By Name(cluster=w369, "State"=State_Enum."Idle") -> (w372:T13)
                n135 = call-poly "Enqueue Message.vi"("error in (no error)"=w367, "Message"="Logging Stopped", "Message Queue"=w374) -> ("error out"=w370:errorcluster)  [unwired: 7 in, 1 out]
              }
              frame "Idle" {
                # "The system is already idle. Ignore the \"Stop\" message."
              }
            }
            n136 = call "Update if Clear.vi"("error in (no error)"=w354, "Message Data"=w359, "Queue in"=w360) -> ("error out"=w356:errorcluster)  [unwired: 8 in]
            n137 = call "Update if Clear.vi"("error in (no error)"=w356, "Message Data"=w357, "Queue in"=w358) -> ("error out"=w355:errorcluster)  [unwired: 8 in]
          }
          frame "Pause" {
            # "Stop - Flush the message queue of any pending \"Log\" messages. Call 'Flush Data to Log File.vi' so any pending data is not lost."
            n138 = Unbundle By Name(w386) -> ("State"=w387:T9, "First Iteration"=w385:bool)
            n139 = case shown="True" w385 {
              tunnel: w386 -> [w390 w395]
              tunnel: [w390 w396] -> w382
              tunnel: w384 -> [w389 w393]
              tunnel: [w389 w392] -> w383
              frame False {
              }
              frame True {
                # "If we load to a paused state we initialize"
                n140 = call "Initialize.vi"("error in (no error)"=w393, "State in"=w395) -> ("error out"=w392:errorcluster, "Pump Initialized"=w397:bool, "State out"=w394:T13)  [unwired: 7 in]
                n141 = case shown="False" w397 {
                  tunnel: [enum16{"Off", "On", "Not Initialized"}."Not Initialized" ("Pump On?") enum16{"Off", "On", "Not Initialized"}."Off" ("Pump On?")] -> w398
                  tunnel: [TRUE FALSE] -> w391
                  frame False {
                  }
                  frame True {
                  }
                }
                n142 = Bundle By Name(cluster=w394, "Pump On?"=w398, "First Iteration"=w391) -> (w396:T13)
              }
            }
            n143 = case shown="\"Measuring\", Default" w387 {
              tunnel: [w407 w415 w419] -> w378
              tunnel: w383 -> [w405 w415 w419]
              tunnel: w388 -> [w411 _ _]
              tunnel: w382 -> [w406 w413 w417]
              tunnel: [w409 w412 w416] -> w381
              frame "Measuring", Default {
                # "If the system is logging, stop logging."
                n144 = call "Pause.vi"("error in (no error)"=w405, "State in"=w406) -> ("error out"=w404:errorcluster, "State out"=w403:T13)  [unwired: 8 in]
                n145 = Bundle By Name(cluster=w403, "State"=State_Enum."Paused") -> (w409:T13)
                n146 = call-poly "Enqueue Message.vi"("error in (no error)"=w404, "Message"="Logging Stopped", "Message Queue"=w411) -> ("error out"=w407:errorcluster)  [unwired: 7 in, 1 out]
              }
              frame "Idle" {
                # "The system is already idle. Ignore the \"Stop\" message."
                n147 = Bundle By Name(cluster=w413, "State"=State_Enum."Paused") -> (w412:T13)
              }
              frame "Paused" {
                n148 = Bundle By Name(cluster=w417, "State"=State_Enum."Paused") -> (w416:T13)
              }
            }
            n149 = call "Update if Clear.vi"("error in (no error)"=w378, "Message Data"=w379, "Queue in"=w380) -> ("error out"=w377:errorcluster)  [unwired: 8 in]
          }
          frame "Update Settings" {
            # "New settings are available, update the current ones stored in the shift register with the settings sent as part of the message"
            n150 = Variant To Data(error in=w426, type=T10 {"Cycle Period"=500.0, "PID 2 Parameters"={"Input Device"=enum."Default", "Output Device"=enum."Equilibar Pressure Reg", "Setpoint"=0.0, "PID gains"={"proportional gain (Kc)"=1.0, "integral time (Ti, min)"=0.01, "derivative time (Td, min)"=0.0}, "output range"={"output low"=0.0, "output high"=100.0}}, "Manual Entry"=0.0, "Auto?"=TRUE, "4-20mA Input Settings"={"Input Channel "=0}, "4-20mA Out Settings"={"Output DAQ Task"=""}, "Input Channel Tag Name "=""} ("Settings"), Variant=w427) -> (data=w421:T10, error out=w424:errorcluster)
            n151 = Bundle By Name(cluster=w423, "Configuration"=w421) -> (w420:T13)
          }
          frame "Exit" {
            # "Release the Logging queue reference"
            # "Don't check the error out. The UI message queue may have already been released."
            # "Stop the VI"
            # "Exit - Send the Exit message to the UI Message Handler.  Call 'Flush Data to Log File.vi' so any pending data is not lost."
            n152 = Release Queue(queue=w432, error in (no error)=w435) -> (error out=w431:errorcluster)  [unwired: 1 in, 2 out]
            n153 = call-poly "Enqueue Message.vi"("Priority Message? (F)"=TRUE, "Message"="Exit", "Message Queue"=w436) -> ("error out"=w430:errorcluster)  [unwired: 7 in, 1 out]
            n154 = call <vilib>:"Clear Errors.vi"("error in (no error)"=w430) -> ()  [unwired: 5 in, 2 out]
            n155 = Merge Errors(w431) -> (w437:errorcluster)
          }
          frame "---Copy This Frame---" {
            # "Duplicate this frame when creating new messages.  Change this comment in the duplicated frame to describe this message."
            n156 = Merge Errors(w442) -> (w441:errorcluster)
          }
          frame Default {
            # "'Default' case only runs if there is a message that isn't defined in any of the other cases.  Output a programming error."
            n157 = Concatenate Strings("The invalid message string " ("string"), w447, " was received in 4-20mA Engine" ("string")) -> (w444:string)
            n158 = Bundle By Name(cluster=errorcluster {"status"=TRUE, "code"=1, "source"=""} ("error constant"), "source"=w444) -> (w443:errorcluster)
          }
        }
        n159 = Unbundle By Name(w17) -> ("State"=w31:T9, "Configuration.Cycle Period"=w29:dbl)
        n160 = call "Error Handler.vi"("error in (no error)"=w37, "Message Queue"=w35) -> ("dup error in"=w36:errorcluster)  [unwired: 8 in, 1 out]
        n161 = case shown="\"Paused\"" w31 {
          tunnel: [w43 1 1] -> w30
          tunnel: w29 -> [w43 _ _]
          frame "Measuring" {
          }
          frame "Idle" {
          }
          frame "Paused" {
          }
        }
        n162 = node-c288(w30) -> ()  [unwired: 1 in, 1 out]
      }
      n163 = node-c288(w12) -> ()  [unwired: 1 out]
    }
    frame Error {
    }
  }
  "error out" <- w3
